vi "publish -- tests -- 1 -- eventful.vi"(7 "publisher action":T1, 10 "stepper pos IN":dbl=1000.0 format="%#_10f") -> (0 "request event":refnum<user-event>, 1 "response event":refnum<user-event>, 2 "stepper pos OUT":dbl=1000.0 format="%#_10f", 4 "response type":dbl)   [LabVIEW 2018]
uses:
  publisher action.ctl
  publisher message -- request.ctl
  publisher message.ctl
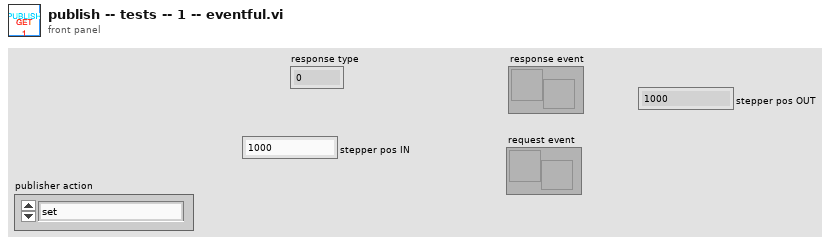
[diagram p1: front panel]
types:
  T1 = typedef "publisher action.ctl" = enum16{"set", "get", "init", "check"}
  T2 = typedef "publisher message.ctl" = cluster{"action":enum16{"next?", "ok"}, "data":dbl}
  T3 = typedef "publisher message -- request.ctl" = cluster{"message action":enum16{"next?", "ok"}}
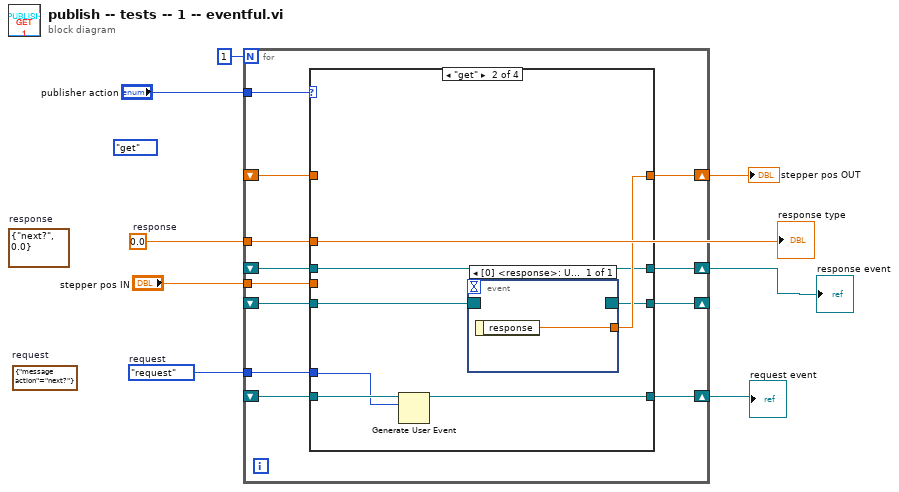
[diagram p0: block diagram]
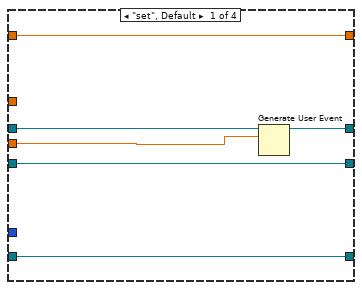
[diagram p2: hidden frame]
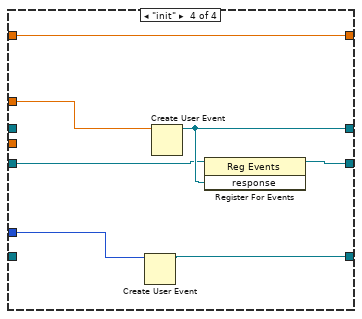
[diagram p4: hidden frame]
diagram:
  w3 = 0.0  # response
  w4 = enum16{"request"}."request"  # request
  (unwired) T2 {"action"=enum."next?", "data"=0.0}  # response
  (unwired) T3 {"message action"=enum."next?"}  # request
  (unwired) publisher_action."get" ("publisher action")
  n1 = for {
    N: 1 -> [_]
    tunnel: "publisher action" -> [w20]
    tunnel: "stepper pos IN" -> [w18]
    shift-right: [w19] -> w5
    shift-left: _ -> [w17]
    shift-right: [w9] -> w1
    shift-left: _ -> [w16]
    shift-right: [w10] -> w2
    shift-left: _ -> [w15]
    shift-right: [w14] -> _
    shift-left: _ -> [w13]
    tunnel: w4 -> [w12]
    tunnel: w3 -> [w11]
    n2 = case shown="\"get\"" w20 {
      tunnel: [w26 w33 w38 w45] -> w19
      tunnel: w18 -> [w23 _ _ _]
      tunnel: w17 -> [w26 _ w38 w45]
      tunnel: w16 -> [w25 w27 w35 _]
      tunnel: w15 -> [w22 w30 w36 _]
      tunnel: [w24 w32 w37 w40] -> w14
      tunnel: w13 -> [w24 w31 w37 w39]
      tunnel: w12 -> [_ w29 _ w43]
      tunnel: w11 -> [_ _ _ w44]
      tunnel: [w22 w28 w36 w42] -> w10
      tunnel: [w21 w27 w35 w41] -> w9
      frame "set", Default {
        n3 = Generate User Event(user event=w25, event data cluster=w23) -> (user event out=w21:refnum<user-event>)  [unwired: 2 in, 1 out]
      }
      frame "get" {
        n4 = Generate User Event(user event=w30, event data cluster=w29) -> (user event out=w28:refnum<user-event>)  [unwired: 2 in, 1 out]
        n5 = event shown="[0] <response>: User Event" {
          selector: w31 -> [_]
          dyn-events: [_] -> w32
          timeout: _ -> [_]
          tunnel: [w34] -> w33
          event User Event {
            n6 = event-data() -> ("response"=w34:dbl)  [unwired: 1 in]
          }
        }
      }
      frame "check" {
      }
      frame "init" {
        n7 = Create User Event(user event datatype=w43) -> (user event=w42:refnum<user-event>)  [unwired: 1 in, 1 out]
        n8 = Create User Event(user event datatype=w44) -> (user event=w41:refnum<user-event>)  [unwired: 1 in, 1 out]
        n9 = register-events(reference=w39, w41) -> (reference out=w40:refnum<event-registration>)  [unwired: 1 in, 1 out]
      }
    }
  }
  "stepper pos OUT" <- w5
  "response event" <- w1
  "request event" <- w2
  "response type" <- w3
